vi "Release.vi"(8 "error in (no error)":errorcluster, 11 "Unsubscribe JSON in":refnum<class "Unsubscribe JSON.lvclass">) -> (0 "error out":errorcluster)   [LabVIEW 2020, in "wamplv.lvlib" / "Unsubscribe JSON.lvclass"]
uses:
  Unsubscribe JSON.lvclass
  Unsubscribe JSON.lvclass/Unsubscribe JSON.ctl
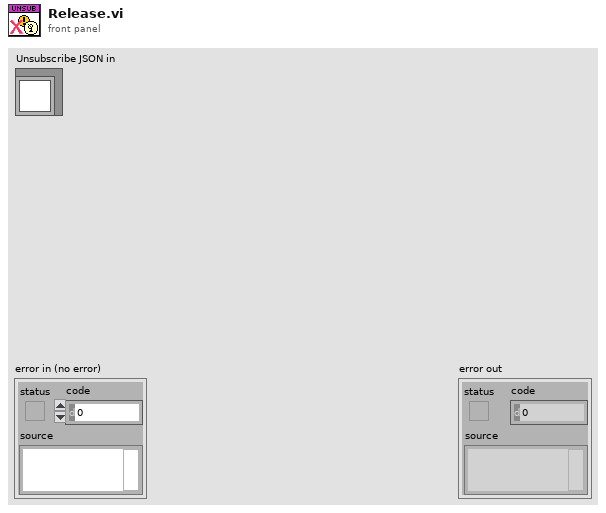
[diagram p1: front panel]
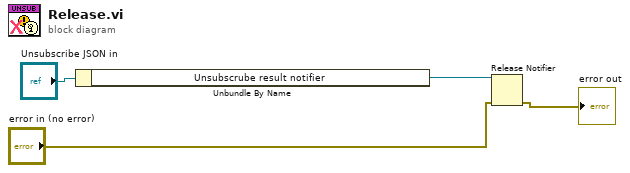
[diagram p0: block diagram]
diagram:
  n1 = Unbundle By Name("Unsubscribe JSON in") -> ("Unsubscrube result notifier"=w3:refnum<notifier>)
  n2 = Release Notifier(notifier=w3, error in (no error)="error in (no error)") -> (error out=→"error out":errorcluster)  [unwired: 1 in, 2 out]
